vi "Read Cycle Time (ms).vi"(8 "error in (no error)":errorcluster, 11 "Multiple Queries in":refnum<class "Multiple Queries.lvclass">) -> (0 "error out":errorcluster, 2 "Cycle Time (ms)":u32, 3 "Multiple Queries out":refnum<class "Multiple Queries.lvclass">)   [LabVIEW 2018, in "Multiple Queries.lvclass"]
doc: "Single Query.lvclass:Read Cycle Time.vi\n\nThis VI is the data accessor for Cycle Time for the Query class.\n\nInstrument Communication Module Version 1.0\nDecember, 2017 Original Code Consulting David Thomson\n www.originalcode.com"
uses:
  Multiple Queries.lvclass
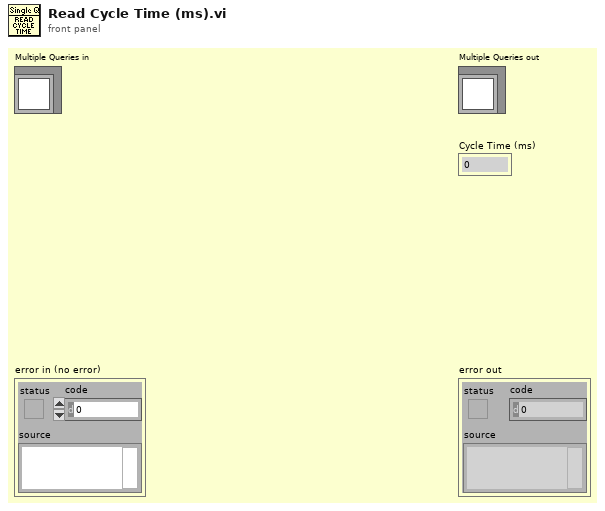
[diagram p1: front panel]
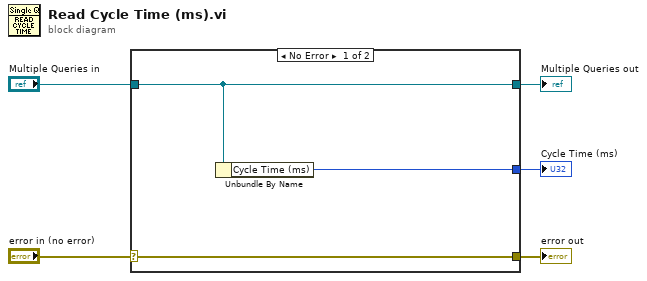
[diagram p0: block diagram]
diagram:
  n1 = case shown="No Error" "error in (no error)" {
    selector: "error in (no error)" -> [w8 w9]
    tunnel: [w8 w9] -> w4
    tunnel: [w7 w10] -> w2
    tunnel: "Multiple Queries in" -> [w7 w10]
    tunnel: [w6 _] -> w1
    frame No Error {
      n2 = Unbundle By Name(w7) -> ("Cycle Time (ms)"=w6:u32)
    }
    frame Error {
    }
  }
  "error out" <- w4
  "Multiple Queries out" <- w2
  "Cycle Time (ms)" <- w1
